vi "Add Attribute Double.vi"(8 "error in (no error)":errorcluster, 9 "data":dbl[](array[numeric]), 10 "Attribute name":string, 11 "loc_id":i32) -> (0 "error out":errorcluster, 3 "loc_id_out":i32)   [LabVIEW 2014, in "HDF5Tools.lvlib"]
uses:
  HDF5Tools.lvlib
  Release/hdf5_hl.dll
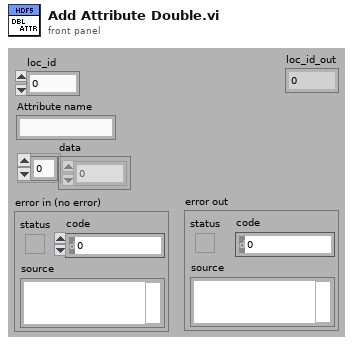
[diagram p1: front panel]
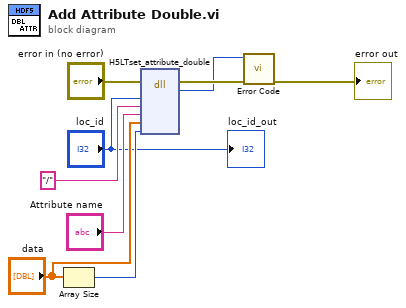
[diagram p0: block diagram]
diagram:
  n1 = Array Size(array="data") -> (size(s)=w5:i32)
  n2 = dll-call lib="Z:/users/Manolis/Labview/Cajal/private/HDF5Tools32/Release/hdf5_hl.dll" fn="H5LTset_attribute_double"(error in="error in (no error)", "loc_id"="loc_id", "obj_name"="/", "attr_name"="Attribute name", "data"="data", "size"=w5) -> (error out=w4:errorcluster, "error"=w2:i32)  [unwired: 7 in, 1 out]
  n3 = call "Error Code.vi"("Error in"=w4, "Error code"=w2) -> ("Error out"=→"error out":errorcluster)  [unwired: 9 in]
  "loc_id_out" <- "loc_id"
